vi "getStatus.vi"(8 "error in (no error)":errorcluster, 11 "StationKeeping in":refnum<class "StationKeeping.lvclass">) -> (0 "error out":errorcluster, 2 "Status":string, 3 "StationKeeping out":refnum<class "StationKeeping.lvclass">)   [LabVIEW 2011, in "StationKeeping.lvclass"]
uses:
  StationKeeping.lvclass
  StationKeeping.lvclass/StationKeeping.ctl
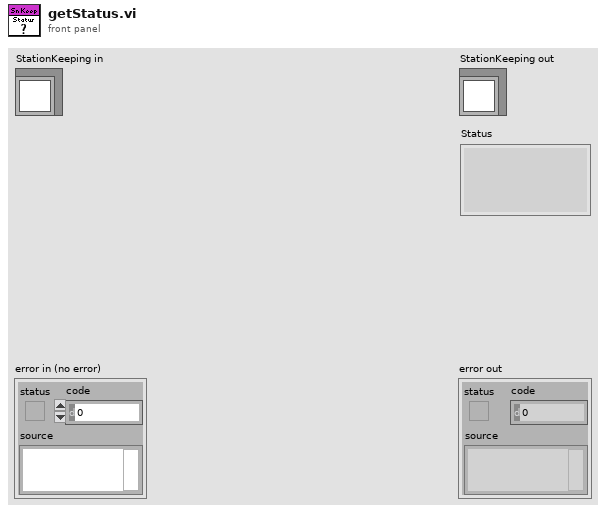
[diagram p1: front panel]
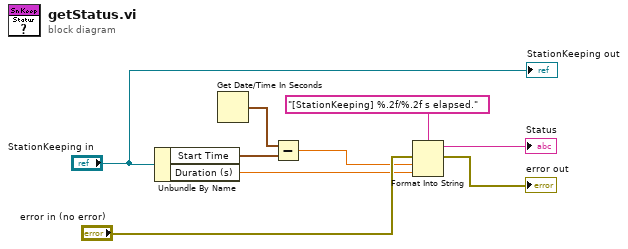
[diagram p0: block diagram]
diagram:
  n1 = Unbundle By Name("StationKeeping in") -> ("Start Time"=w8:timestamp, "Duration (s)"=w4:dbl)
  n2 = Get Date/Time In Seconds() -> (seconds since 1Jan1904=w9:timestamp)
  n3 = Subtract(x=w9, y=w8) -> (x-y=w1:dbl)
  n4 = Format Into String(format string="[StationKeeping] %.2f/%.2f s elapsed.", error in="error in (no error)", w1, w4) -> (resulting string=→"Status":string, error out=→"error out":errorcluster)  [unwired: 1 in]
  "StationKeeping out" <- "StationKeeping in"
